vi "textInteractionFlags.vi"(8 "Error In":errorcluster, 11 "QMessageBox In":refnum<class "QMessageBox.lvclass">) -> (0 "Error Out":errorcluster, 2 "Value":T1 items=["NoTextInteraction"=0, "TextSelectableByMouse"=1, "TextSelectableByKeyboard"=2, "LinksAccessibleByMouse"=4, "LinksAccessibleByKeyboard"=8, "TextEditable"=16, "TextEditorInteraction"=19, "TextBrowserInteraction"=13], 3 "QMessageBox Out":refnum<class "QMessageBox.lvclass">)   [LabVIEW 2014, in "QMessageBox.lvclass"]
doc: "LabVIEW-specific documentation is not yet available. See <b>https://doc.qt.io/qt-5/qmessagebox.html#textInteractionFlags</b>"
uses:
  QMessageBox.lvclass
  LQ Core/Qt/TextInteractionFlag.ctl
  LQ Core/LQIdentity/LQIdentity.lvclass/LQIdentity.ctl
  LQ Core/LQ Core.lvlib
  LQ Core/LQIdentity/LQIdentity.lvclass
  LQ Core/Qt/Qt.lvlib
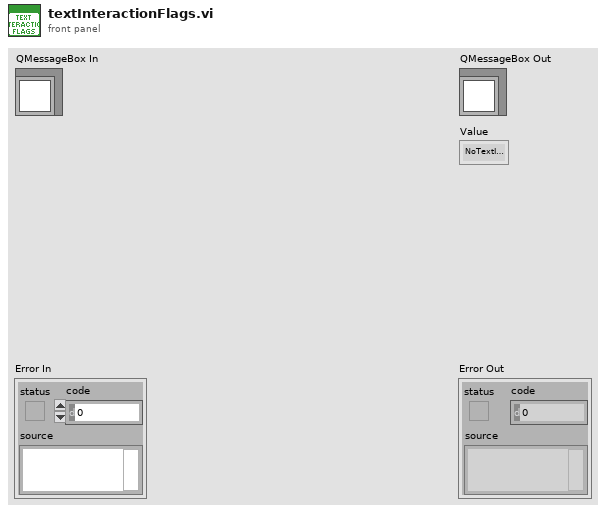
[diagram p1: front panel]
types:
  T1 = typedef "Qt.lvlib/TextInteractionFlag.ctl" = i32
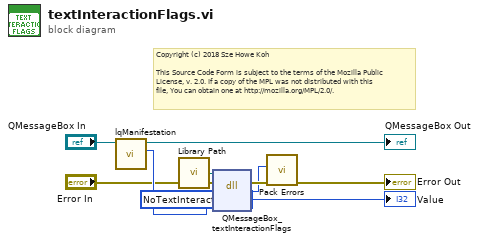
[diagram p0: block diagram]
diagram:
  w7 = T1 0 items=["NoTextInteraction"=0, "TextSelectableByMouse"=1, "TextSelectableByKeyboard"=2, "LinksAccessibleByMouse"=4, "LinksAccessibleByKeyboard"=8, "TextEditable"=16, "TextEditorInteraction"=19, "TextBrowserInteraction"=13] ("retVal")
  # "Copyright (c) 2018 Sze Howe Koh\n\nThis Source Code Form is subject to the terms of the Mozilla Public\nLicense, v. 2.0. If a copy of the MPL was not distributed with this\nfile, You can obtain one at http://mozilla.org/MPL/2.0/."
  n1 = call "lqManifestation.vi"("LQIdentity in"="QMessageBox In") -> ("Manifestation"=w5:u64, "LQIdentity out"=→"QMessageBox Out":refnum<class "QMessageBox.lvclass">)  [unwired: 9 in]
  n2 = call "Library Path.vi"() -> ("Library Path"=w6:path)
  n3 = dll-call lib="?" fn="QMessageBox_textInteractionFlags"(path in=w6, error in="Error In", "_retVal"=w7, "_instance"=w5) -> (error out=w3:errorcluster, w1:i32, "_retVal"=→"Value":i32)  [unwired: 2 in, 1 out]
  n4 = call "Pack Errors.vi"("Error In"=w3, "Error Code"=w1) -> ("Error Out"=→"Error Out":errorcluster)  [unwired: 9 in]
